vi "Auto 7.vi"(8 "Error In":errorcluster) -> (0 "Error Out":errorcluster)   [LabVIEW 2014]
uses:
  <vilib>/Rock Robotics/WPI/Solenoid/WPI_SolenoidValue.ctl
  <vilib>/Rock Robotics/WPI/Solenoid/WPI_SolenoidSetEnum.vi
  <vilib>/Rock Robotics/Network Tables/SD Read Boolean.vi
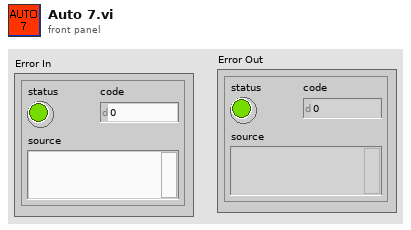
[diagram p1: front panel]
types:
  T1 = typedef "WPI_SolenoidValue.ctl" = enum16{"Off", "On", "Forward", "Reverse"}
  T2 = typedef "WPI_SolenoidDevRef.ctl" = cluster{"DevStatus":errorcluster, "Pneumatics Control Module":u8, "Forward Solenoid Channel":T3, "Reverse Solenoid Channel":T3}
  T3 = typedef "WPI_SolenoidChannel.ctl" = enum8{"Solenoid 0", "Solenoid 1", "Solenoid 2", "Solenoid 3", "Solenoid 4", "Solenoid 5", "Solenoid 6", "Solenoid 7", "Invalid"}
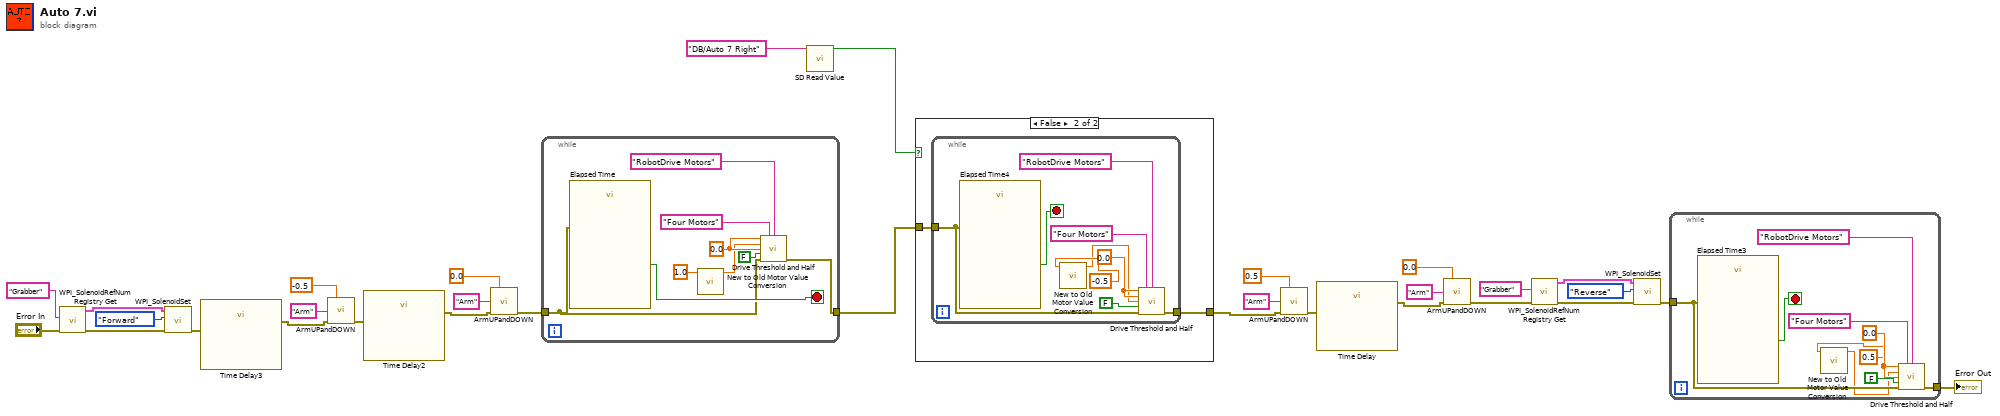
[diagram p0: block diagram]
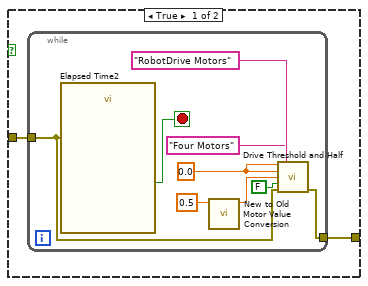
[diagram p2: hidden frame]
diagram:
  n1 = call <vilib>:"WPI_SolenoidRefNum Registry Get.vi"("error in (no error)"="Error In", "refnum name"="Grabber") -> ("error out"=w18:errorcluster, "SolenoidDevRef"=w19:T2)  [unwired: 8 in]
  n2 = call-poly <vilib>:"WPI_SolenoidSet.vi"("error in (no error)"=w18, "Value"=WPI_SolenoidValue."Forward", "SolenoidDevRef"=w19) -> ("error out"=w7:errorcluster)  [unwired: 7 in, 1 out]
  n3 = call "Time Delay3"("error in (no error)"=w7) -> ("error out"=w6:errorcluster)  [unwired: 10 in]
  n4 = call "ArmUPandDOWN.vi"("Arm Value"=-0.5, "Arm"="Arm" ("refnum name"), "Error In"=w6) -> ("Error Out"=w29:errorcluster)  [unwired: 12 in]
  n5 = call "Time Delay2"("error in (no error)"=w29) -> ("error out"=w12:errorcluster)  [unwired: 10 in]
  n6 = call "ArmUPandDOWN.vi"("Arm Value"=0.0, "Arm"="Arm" ("refnum name"), "Error In"=w12) -> ("Error Out"=w5:errorcluster)  [unwired: 12 in]
  n7 = while {
    tunnel: w5 -> [w34]
    tunnel: [w37] -> w1
    stop <- w35 stop-if-true
    w36 = 0.0 ("Arm Value")
    n8 = call "Elapsed Time"("error in (no error)"=w34) -> ("Time has Elapsed"=w35:bool)  [unwired: 11 in, 7 out]
    n9 = call "New to Old Motor Value Conversion.vi"("Motor Value In"=1.0 ("X In")) -> ("New to Old Conversion Value Out"=w32:dbl)  [unwired: 9 in, 1 out]
    n10 = call "Drive Threshold and Half.vi"("X In"=w36, "Drive refnum name"="Four Motors" ("refnum name"), "Send to DB Name"="RobotDrive Motors" ("Name"), "Y In"=w32, "R In"=w36, "Speed Toggle"=FALSE ("Grabber Open/Close"), "Error In"=w34) -> ("Error Out"=w37:errorcluster)  [unwired: 8 in]
  }
  n11 = call-poly <vilib>:"SD Read Value.vi"("Name"="DB/Auto 7 Right") -> ("Boolean"=w3:bool)  [unwired: 8 in, 2 out]
  n12 = case shown="False" w3 {
    tunnel: w1 -> [w42 w53]
    tunnel: [w41 w52] -> w2
    frame True {
      n13 = while {
        tunnel: w42 -> [w45]
        tunnel: [w48] -> w41
        stop <- w46 stop-if-true
        w47 = 0.0 ("Arm Value")
        n14 = call "Elapsed Time2"("error in (no error)"=w45) -> ("Time has Elapsed"=w46:bool)  [unwired: 11 in, 7 out]
        n15 = call "New to Old Motor Value Conversion.vi"("Motor Value In"=0.5 ("X In")) -> ("New to Old Conversion Value Out"=w43:dbl)  [unwired: 9 in, 1 out]
        n16 = call "Drive Threshold and Half.vi"("X In"=w47, "Drive refnum name"="Four Motors" ("refnum name"), "Send to DB Name"="RobotDrive Motors" ("Name"), "Y In"=w47, "R In"=w43, "Speed Toggle"=FALSE ("Grabber Open/Close"), "Error In"=w45) -> ("Error Out"=w48:errorcluster)  [unwired: 8 in]
      }
    }
    frame False {
      n17 = while {
        tunnel: w53 -> [w56]
        tunnel: [w58] -> w52
        stop <- w57 stop-if-true
        w59 = 0.0 ("Arm Value")
        n18 = call "Elapsed Time4"("error in (no error)"=w56) -> ("Time has Elapsed"=w57:bool)  [unwired: 11 in, 7 out]
        n19 = call "New to Old Motor Value Conversion.vi"("Motor Value In"=-0.5 ("X In")) -> ("New to Old Conversion Value Out"=w54:dbl)  [unwired: 9 in, 1 out]
        n20 = call "Drive Threshold and Half.vi"("X In"=w59, "Drive refnum name"="Four Motors" ("refnum name"), "Send to DB Name"="RobotDrive Motors" ("Name"), "Y In"=w59, "R In"=w54, "Speed Toggle"=FALSE ("Grabber Open/Close"), "Error In"=w56) -> ("Error Out"=w58:errorcluster)  [unwired: 8 in]
      }
    }
  }
  n21 = call "ArmUPandDOWN.vi"("Arm Value"=0.5, "Arm"="Arm" ("refnum name"), "Error In"=w2) -> ("Error Out"=w27:errorcluster)  [unwired: 12 in]
  n22 = call "Time Delay"("error in (no error)"=w27) -> ("error out"=w9:errorcluster)  [unwired: 10 in]
  n23 = call "ArmUPandDOWN.vi"("Arm Value"=0.0, "Arm"="Arm" ("refnum name"), "Error In"=w9) -> ("Error Out"=w8:errorcluster)  [unwired: 12 in]
  n24 = call <vilib>:"WPI_SolenoidRefNum Registry Get.vi"("error in (no error)"=w8, "refnum name"="Grabber") -> ("error out"=w23:errorcluster, "SolenoidDevRef"=w24:T2)  [unwired: 8 in]
  n25 = call-poly <vilib>:"WPI_SolenoidSet.vi"("error in (no error)"=w23, "Value"=WPI_SolenoidValue."Reverse", "SolenoidDevRef"=w24) -> ("error out"=w20:errorcluster)  [unwired: 7 in, 1 out]
  n26 = while {
    tunnel: w20 -> [w65]
    tunnel: [w68] -> w28
    stop <- w66 stop-if-true
    w67 = 0.0 ("Arm Value")
    n27 = call "Elapsed Time3"("error in (no error)"=w65) -> ("Time has Elapsed"=w66:bool)  [unwired: 11 in, 7 out]
    n28 = call "New to Old Motor Value Conversion.vi"("Motor Value In"=0.5 ("X In")) -> ("New to Old Conversion Value Out"=w63:dbl)  [unwired: 9 in, 1 out]
    n29 = call "Drive Threshold and Half.vi"("X In"=w67, "Drive refnum name"="Four Motors" ("refnum name"), "Send to DB Name"="RobotDrive Motors" ("Name"), "Y In"=w63, "R In"=w67, "Speed Toggle"=FALSE ("Grabber Open/Close"), "Error In"=w65) -> ("Error Out"=w68:errorcluster)  [unwired: 8 in]
  }
  "Error Out" <- w28
